vi "Timing_GCFS.vi"(0 "?":T1={"Core"={"Current VI Reference"=refnum, "Close Panel on Exit?"=FALSE}, "Camera Cluster"={"Session"="", "Image"=refnum, "Position Image"=refnum, "PixelVal Image"=refnum, "Position Image Binary"=refnum, "Lable Image"=refnum, "Merged Image"=refnum, "Connection"=FALSE}, "Data In Cluster"={"Images"={"Position Image path"=path "", "Sample folder path"=path "", "Label Image path"=path ""}, "Sample Name"="", "Sample Rate"=0, "Gradient Buffer"=0, "Data Acquisition.Setup.TempGrad"=0.0, "Control.PID gains"={"proportional gain (Kc)"=0.0, "integral time (Ti, min)"=0.0, "derivative time (Td, min)"=0.0}, "Freezing value"=250.0, "Sample Rate 2"=20}, "Active"=FALSE, "Ready"=FALSE, "Exit"=FALSE, "Arduino"={"Connection"=FALSE, "Port"="", "State"=""}, "Program_Start"="", "Data Out Cluster"={"Particle Measurements"=[], "Number of droplets"=0, "PosImg_Timestamp"="", "OverlayProp"=[], "Group"="", "Que"=refnum}, "PSU"={"Connection"=FALSE, "Port"="", "State"=""}, "Load Rerun"=FALSE, "Rerun"=FALSE, "cDAQ"={"Connection"=FALSE, "ID"="", "Task"=""}, "Temp"={"Manual Temp"=FALSE, "Target"=0.0}, "Cool A."=FALSE} {"Data Out Cluster"."Particle Measurements" format="%.2f"; "Data In Cluster"."Sample Rate 2" min=20 max=240 format="%.0f samples/min"}) -> (1 "Sample dt (ms)":i64, 2 "Sample dt (s)":dbl)   [LabVIEW 2024]
uses:
  Micro/DataCluster_GCFS.ctl
  <vilib>/userDefined/High Color/IMAQdx.ctl
  <vilib>/vision/Image Controls.llb/IMAQ Image.ctl
  <vilib>/vision/Image Controls.llb/Overlay Property.ctl
panel:
  # "2,6 On INC_Old"
  # "0,08 On INC_Old"
  # "0,1 On INC_Old"
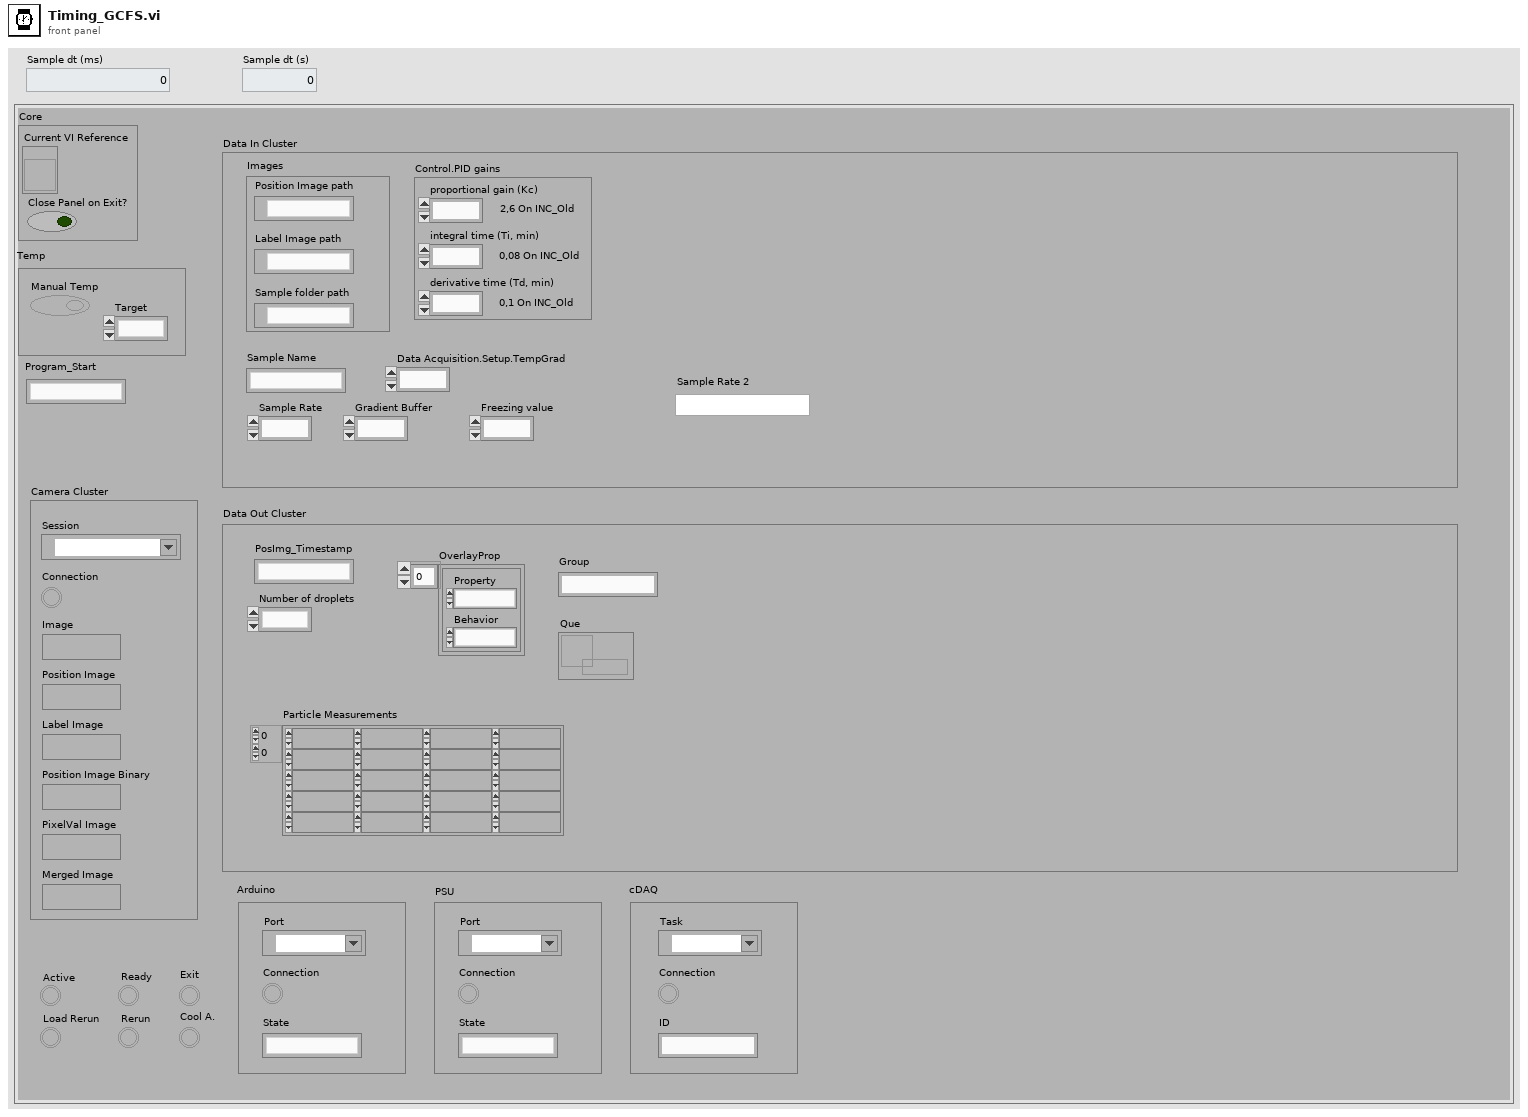
[diagram p1: front panel]
types:
  T1 = typedef "DataCluster_GCFS.ctl" = cluster{"Core":cluster{"Current VI Reference":refnum<vi>, "Close Panel on Exit?":bool}, "Camera Cluster":cluster{"Session":T2, "Image":T3, "Position Image":T3, "PixelVal Image":T3, "Position Image Binary":T3, "Lable Image":T3, "Merged Image":T3, "Connection":bool}, "Data In Cluster":cluster{"Images":cluster{"Position Image path":path, "Sample folder path":path, "Label Image path":path}, "Sample Name":string, "Sample Rate":i32, "Gradient Buffer":i32, "Data Acquisition.Setup.TempGrad":dbl, "Control.PID gains":cluster{"proportional gain (Kc)":dbl, "integral time (Ti, min)":dbl, "derivative time (Td, min)":dbl}, "Freezing value":sgl, "Sample Rate 2":i32}, "Active":bool, "Ready":bool, "Exit":bool, "Arduino":cluster{"Connection":bool, "Port":refnum<visa-resource-name>, "State":string}, "Program_Start":string, "Data Out Cluster":cluster{"Particle Measurements":dbl[][], "Number of droplets":i32, "PosImg_Timestamp":string, "OverlayProp":T4[], "Group":string, "Que":refnum<queue>}, "PSU":cluster{"Connection":bool, "Port":refnum<visa-resource-name>, "State":string}, "Load Rerun":bool, "Rerun":bool, "cDAQ":cluster{"Connection":bool, "ID":string, "Task":refnum<k21>}, "Temp":cluster{"Manual Temp":bool, "Target":dbl}, "Cool A.":bool}
  T2 = typedef "IMAQdx.ctl" = refnum<k21>
  T3 = typedef "IMAQ Image.ctl" = refnum<image>
  T4 = typedef "Overlay Property.ctl" = cluster{"Property":enum32{"Scale", "Shift", "Rotate", "Symmetry"}, "Behavior":enum32{"Clear", "Keep", "Transform"}}
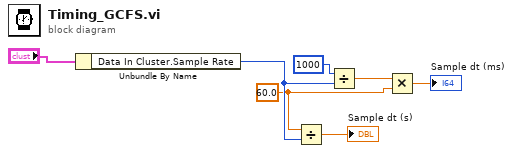
[diagram p0: block diagram]
diagram:
  w4 = 60.0 ("y")
  n1 = Unbundle By Name("?") -> ("Data In Cluster.Sample Rate"=w5:i32)
  n2 = Divide(x=w4, y=w5) -> (x/y=→"Sample dt (s)":dbl)
  n3 = Divide(x=1000, y=w5) -> (x/y=w1:dbl)
  n4 = Multiply(x=w1, y=w4) -> (x*y=→"Sample dt (ms)":dbl)
